vi "interview.vi"(0 "HB_PollingAgent in":refnum<class "HB_PollingAgent.lvclass">, 11 "error in (no error)":errorcluster) -> (4 "HB_PollingAgent out":refnum<class "HB_PollingAgent.lvclass">, 15 "error out":errorcluster)   [LabVIEW 2009, in "HB_PollingAgent.lvlib" / "HB_PollingAgent.lvclass"]
uses:
  HB_PollingAgent.lvclass
  HB_PollingAgent.lvclass/HB_PollingAgent.ctl
  lib.lib/HGF_LVC/HGF_MobileAgentSystem/MoAgSy_AgentBase/MoAgSy_AgentBase.lvclass
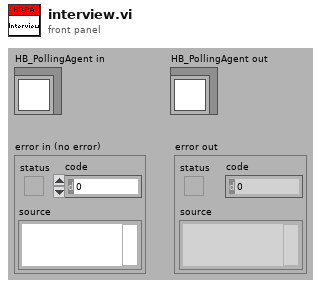
[diagram p1: front panel]
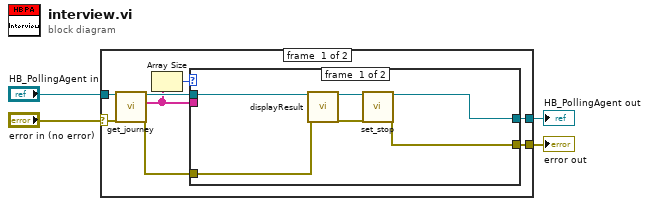
[diagram p0: block diagram]
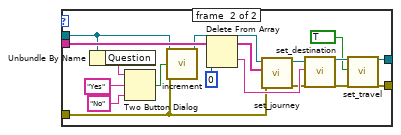
[diagram p2: hidden frame]
diagram:
  n1 = case shown="No Error" "error in (no error)" {
    selector: "error in (no error)" -> [w5 w38]
    tunnel: [w7 w38] -> w3
    tunnel: [w8 w37] -> w1
    tunnel: "HB_PollingAgent in" -> [w6 w37]
    frame #0 {
      n2 = call "get_journey.vi"("HGF_Agent in"=w6, "error in (no error)"=w5) -> ("HGF_Agent out"=w12:refnum<class "HB_PollingAgent.lvclass">, "journey"=w10:string[], "error out"=w9:errorcluster)  [unwired: 15 in]
      n3 = Array Size(array=w10) -> (size(s)=w11:i32)
      n4 = case shown="Default" w11 {
        tunnel: w12 -> [w16 w20]
        tunnel: [w18 w36] -> w8
        tunnel: w10 -> [_ w35]
        tunnel: w9 -> [w15 w21]
        tunnel: [w17 w27] -> w7
        frame #0 {
          n5 = call "displayResult.vi"("HB_PollingAgent in"=w16, "error in (no error)"=w15) -> ("HB_PollingAgent out"=w13:refnum<class "HB_PollingAgent.lvclass">, "error out"=w14:errorcluster)  [unwired: 12 in]
          n6 = call "set_stop.vi"("HGF_Agent.lvclass in"=w13, "error in (no error)"=w14) -> ("HGF_Agent.lvclass out"=w18:refnum<class "HB_PollingAgent.lvclass">, "error out"=w17:errorcluster)  [unwired: 16 in]
        }
        frame #1 {
          n7 = Unbundle By Name(w20) -> ("Question"=w22:string)
          n8 = Two Button Dialog(message=w22, 1:"No" ("F button name (\"Cancel\")"), 2:"Yes" ("T button name (\"OK\")")) -> (T button?=w23:bool)
          n9 = call "increment.vi"("HB_PollingAgent in"=w20, "T:Yes,F:No"=w23, "error in (no error)"=w21) -> ("HB_PollingAgent out"=w19:refnum<class "HB_PollingAgent.lvclass">)  [unwired: 11 in, 1 out]
          n10 = Delete From Array(array=w35, index=0) -> (deleted portion=w32:string, array with subset deleted=w33:string[])  [unwired: 1 in]
          n11 = call "set_journey.vi"("error in (no error)"=w21, "journey"=w33, "MoAgSy_AgentBase in"=w19) -> ("error out"=w28:errorcluster, "MoAgSy_AgentBase out"=w31:refnum<class "HB_PollingAgent.lvclass">)  [unwired: 7 in]
          n12 = call "set_destination.vi"("HGF_Agent in"=w31, "destination"=w32, "error in (no error)"=w28) -> ("HGF_Agent out"=w30:refnum<class "HB_PollingAgent.lvclass">, "error out"=w29:errorcluster)  [unwired: 15 in]
          n13 = call "set_travel.vi"("HGF_Agent in"=w30, "travel?"=TRUE, "error in (no error)"=w29) -> ("HGF_Agent out"=w36:refnum<class "HB_PollingAgent.lvclass">, "error out"=w27:errorcluster)  [unwired: 15 in]
        }
      }
    }
    frame #1 {
    }
  }
  "error out" <- w3
  "HB_PollingAgent out" <- w1
